vi "combine2imagesInArray.vi"(8 "Beam in":T1, 11 "Image in":T1) -> (3 "Array":u8[][][](array[numeric]))   [LabVIEW 2022 SP3]
uses:
  <vilib>/vision/Image Controls.llb/IMAQ Image.ctl
  <vilib>/vision/NI_Vision_Development_Module.lvlib
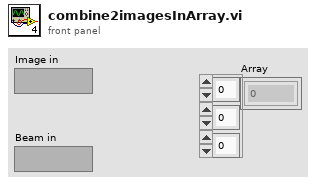
[diagram p1: front panel]
types:
  T1 = typedef "IMAQ Image.ctl" = refnum<image>
  T2 = cluster{"Red (or Hue) value":u8, "Green (or Sat) value":u8, "Blue (or Light or Val) value":u8}
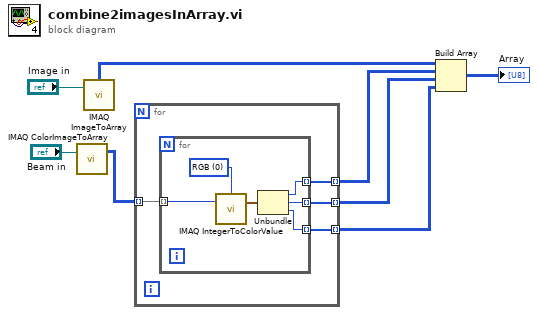
[diagram p0: block diagram]
diagram:
  n1 = call "IMAQ ColorImageToArray"("Image"="Beam in") -> ("Image Pixels (U32)"=w4:u32[][])  [unwired: 3 in, 2 out]
  n2 = call "IMAQ ImageToArray"("Image"="Image in") -> ("Image Pixels (U8)"=w6:u8[][])  [unwired: 3 in, 4 out]
  n3 = for {
    tunnel: w4 -> [w12] mode=indexing
    tunnel: [w11] -> w3 mode=indexing
    tunnel: [w10] -> w2 mode=indexing
    tunnel: [w9] -> w1 mode=indexing
    n4 = for {
      tunnel: w12 -> [w17] mode=indexing
      tunnel: [w15] -> w11 mode=indexing
      tunnel: [w14] -> w10 mode=indexing
      tunnel: [w13] -> w9 mode=indexing
      w18 = u16 0 items=["RGB", "HSL", "HSV", "HSI"] ("Color Mode")
      n5 = call "IMAQ IntegerToColorValue"("U32 value"=w17, "Color Mode"=w18) -> ("Color Value"=w16:T2)  [unwired: 3 in, 3 out]
      n6 = Unbundle(w16) -> ("Red (or Hue) value"=w15:u8, "Green (or Sat) value"=w14:u8, "Blue (or Light or Val) value"=w13:u8)
    }
  }
  n7 = Build Array(w6, w3, w2, w1) -> (→"Array":u8[][][])
